vi "Configure Average.vi"(7 "Average on":bool, 8 "error in (no error)":errorcluster, 10 "Average Count":i32, 11 "U2000 in":refnum<class "U2000.lvclass">) -> (0 "error out":errorcluster, 3 "U2000 out":refnum<class "U2000.lvclass">)   [LabVIEW 2020, in "U2000.lvclass"]
uses:
  U2000.lvclass
  C:/Sandbox/RF Bench/Source Code/WiSpry Test Framework/Instruments/Instrument.lvclass
  C:/Sandbox/RF Bench/Source Code/WiSpry Test Framework/Instruments/Power Meter/Power Meter.lvclass
  Power Meter.lvclass/Power Meter.ctl
  Instrument.lvclass/Instrument.ctl
  <instrlib>/Agilent U2000 Series/Agilent U2000 Series.lvlib
  Instrument.lvclass
  Power Meter.lvclass
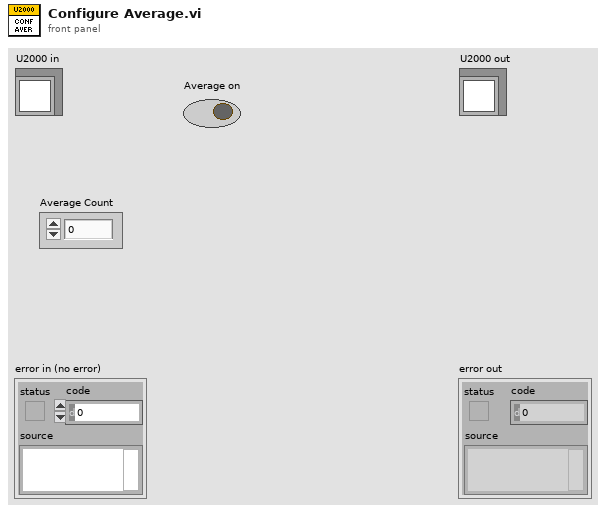
[diagram p1: front panel]
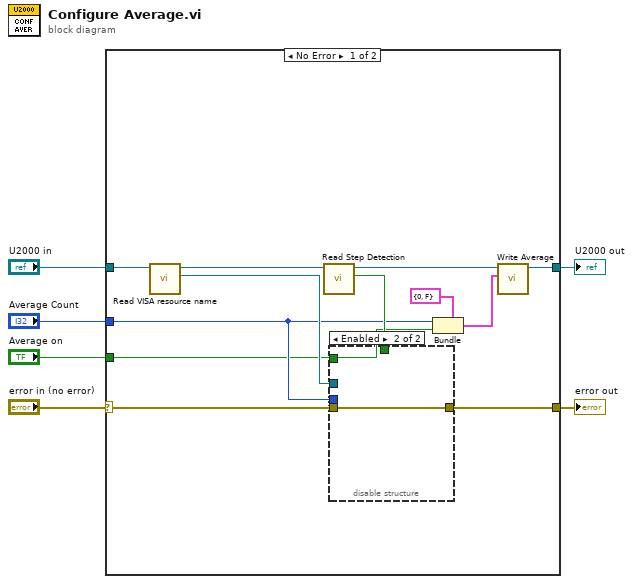
[diagram p0: block diagram]
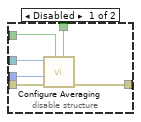
[diagram p2: hidden frame]
diagram:
  n1 = case shown="No Error" "error in (no error)" {
    selector: "error in (no error)" -> [w18 w27]
    tunnel: [w11 w27] -> w5
    tunnel: "Average on" -> [w8 _]
    tunnel: "Average Count" -> [w9 _]
    tunnel: "U2000 in" -> [w17 w26]
    tunnel: [w12 w26] -> w1
    frame No Error {
      n2 = call "Read VISA resource name.vi"("Instrument in"=w17) -> ("VISA resource name"=w16:refnum<visa-resource-name>, "Instrument out"=w15:refnum<class "U2000.lvclass">)  [unwired: 9 in]
      n3 = call "Read Step Detection.vi"("Power Meter in"=w15) -> ("Step Detection"=w14:bool, "Power Meter out"=w13:refnum<class "U2000.lvclass">)  [unwired: 9 in]
      n4 = disable-structure shown="Enabled" {
        disable-tunnel: w18 -> [w24 w25]
        disable-tunnel: w16 -> [w23 _]
        disable-tunnel: w14 -> [w22 _]
        disable-tunnel: [w21 w25] -> w11
        disable-tunnel: w9 -> [w20 _]
        disable-tunnel: w8 -> [w19 _]
        frame Disabled {
          n5 = call <instrlib>:"Configure Averaging.vi"("Enable Step Detection (T: Enable)"=w22, "Enable Averaging (T: Enable)"=w19, "error in (no error)"=w24, "Averaging Count (4)"=w20, "VISA resource name"=w23) -> ("error out"=w21:errorcluster)  [unwired: 5 in, 1 out]
        }
        frame Enabled {
        }
      }
      n6 = Bundle(cluster=cluster{"Average":i32, "Average State":bool} {"Average"=0, "Average State"=FALSE} ("Average"), "Average"=w9, "Average State"=w8) -> (w7:cluster{"Average":i32, "Average State":bool})
      n7 = call "Write Average.vi"("Average"=w7, "Power Meter in"=w13) -> ("Power Meter out"=w12:refnum<class "U2000.lvclass">)  [unwired: 9 in]
    }
    frame Error {
    }
  }
  "error out" <- w5
  "U2000 out" <- w1
